vi "JSON to LVObject.vi"(7 "BlueJSONtext LVClass Serializer in":refnum<class "BlueJSONtext LVClass Serializer.lvclass">, 8 "error in (no error)":errorcluster, 9 "Object Type":refnum<class>, 10 "Offset":i32, 11 "JSON":string) -> (0 "error out":errorcluster, 1 "Object":refnum<class>)   [LabVIEW 2019, in "BlueJSONTextSerializer.lvlib" / "BlueJSONtext LVClass Serializer.lvclass"]
uses:
  BlueJSONtext LVClass Serializer.lvclass
  BlueJSONtext LVClass Serializer.lvclass/BlueJSONtext LVClass Serializer.ctl
  BlueJSONTextSerializer/StructuredData.ctl
  BlueJSONTextSerializer/BlueJSONTextSerializer.lvclass
  C:/Program Files (x86)/National Instruments/LabVIEW 2019/user.lib/Blue Origin/BlueSerialization/BlueSerializer/BlueSerializer.lvclass
  <userlib>/Blue Origin/BlueSerialization/BlueSerializer/BlueSerializer.lvclass
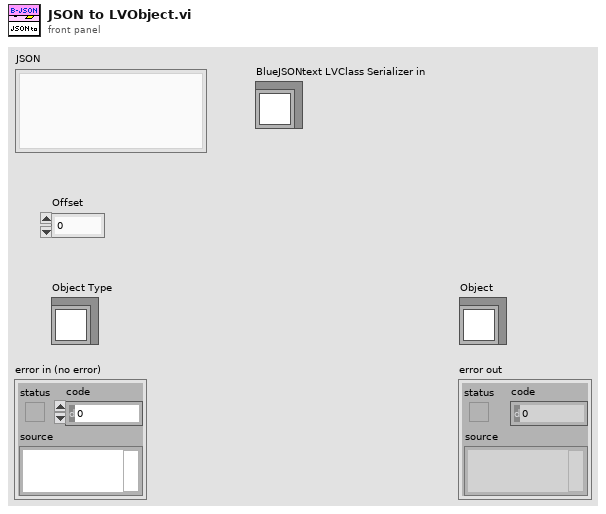
[diagram p1: front panel]
types:
  T1 = typedef "BlueJSONTextSerializer.lvlib/BlueJSONTextSerializer.lvclass/StructuredData.ctl" = cluster{"JSON":string, "Offset":i32}
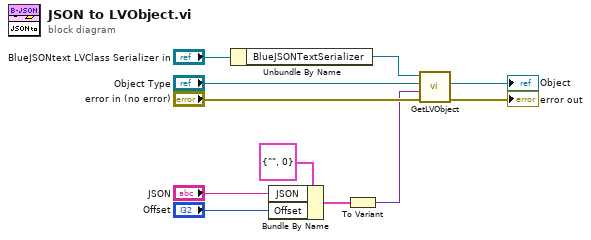
[diagram p0: block diagram]
diagram:
  n1 = Unbundle By Name("BlueJSONtext LVClass Serializer in") -> ("BlueJSONTextSerializer"=w4:refnum<class "BlueJSONTextSerializer.lvclass">)
  n2 = Bundle By Name(cluster=T1 {"JSON"="", "Offset"=0} ("Cluster"), "JSON"="JSON", "Offset"="Offset") -> (w7:T1)
  n3 = To Variant(anything=w7) -> (Variant=w6:variant)
  n4 = call <userlib>:"GetLVObject.vi"("error in (no error)"="error in (no error)", "StructuredData in"=w6, "Object Type"="Object Type", "BlueSerializer in"=w4) -> ("error out"=→"error out":errorcluster, "Object out"=→"Object":refnum<class>)  [unwired: 4 in, 2 out]
